vi "execute.vi"(8 "error in (no error)":errorcluster, 9 "DAQ in":refnum<class "GenericComponent.lvclass">, 10 "imaging mode in":refnum<class "GenericComponent.lvclass">, 11 "AdapterDL091214ImagingModeToDAQ in":refnum<class "AdapterDL091214ImagingModeToDAQ.lvclass">) -> (0 "error out":errorcluster, 1 "DAQ out":refnum<class "GenericComponent.lvclass">, 2 "imaging mode out":refnum<class "GenericComponent.lvclass">, 3 "AdapterDL091214ImagingModeToDAQ out":refnum<class "AdapterDL091214ImagingModeToDAQ.lvclass">)   [LabVIEW 2010, in "AdapterDL091214ImagingModeToDAQ.lvclass"]
uses:
  AdapterDL091214ImagingModeToDAQ.lvclass
  common/classes/GenericComponent/GenericComponent/GenericComponent.lvclass
  DAQ/DAQ_MG090622Camera/DAQ_MG090622Camera/DAQ_MG090622Camera.lvclass
  ImagingMode/ImagingModeMG090624Camera/ImagingModeMG090624Camera/ImagingModeMG090624Camera.lvclass
panel:
  # "ScanMode: ImagingModeMG090624Camera \nDAQ: DAQ_MG090622Camera"
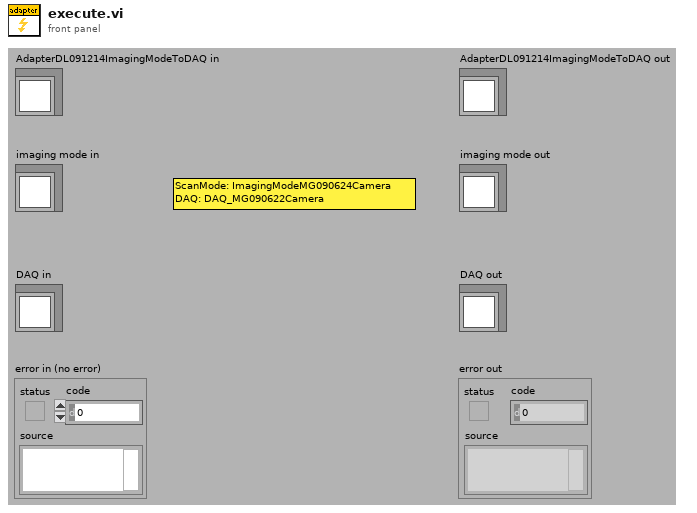
[diagram p1: front panel]
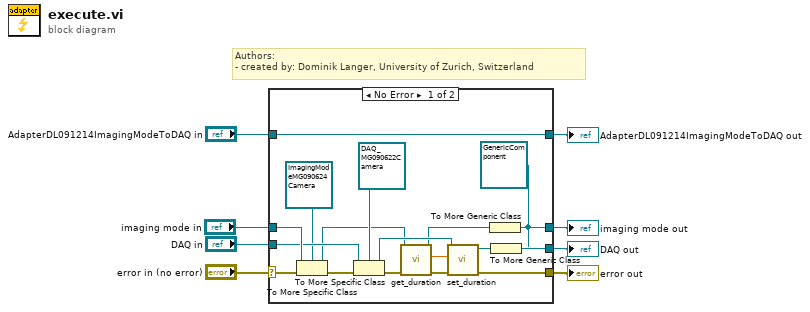
[diagram p0: block diagram]
diagram:
  # "Authors: \n- created by: Dominik Langer, University of Zurich, Switzerland"
  n1 = case shown="No Error" "error in (no error)" {
    selector: "error in (no error)" -> [w25 w29]
    tunnel: "DAQ in" -> [w22 w28]
    tunnel: "imaging mode in" -> [w24 w27]
    tunnel: [w26 w30] -> w4
    tunnel: "AdapterDL091214ImagingModeToDAQ in" -> [w26 w30]
    tunnel: [w16 w29] -> w3
    tunnel: [w19 w28] -> w2
    tunnel: [w17 w27] -> w1
    frame No Error {
      w18 = refnum<class "GenericComponent.lvclass"> refnum ("GenericComponent.lvclass")
      n2 = To More Specific Class(target class=refnum<class "ImagingModeMG090624Camera.lvclass"> refnum ("ImagingModeMG090624Camera.lvclass"), reference=w24, error in=w25) -> (specific class reference=w11:refnum<class "ImagingModeMG090624Camera.lvclass">, error out=w23:errorcluster)
      n3 = To More Specific Class(target class=refnum<class "DAQ_MG090622Camera.lvclass"> refnum ("DAQ_MG090622Camera.lvclass"), reference=w22, error in=w23) -> (specific class reference=w15:refnum<class "DAQ_MG090622Camera.lvclass">, error out=w13:errorcluster)
      n4 = call-dynamic "get_duration.vi"("error in (no error)"=w13, "ScanModeMG090624Camera in"=w11) -> ("error out"=w12:errorcluster, "duration"=w9:dbl[unit], "ScanModeMG090624Camera out"=w10:refnum<class "ImagingModeMG090624Camera.lvclass">)  [unwired: 7 in]
      n5 = call-dynamic "set_duration.vi"("error in (no error)"=w12, "duration"=w9, "DAQ_MG090622Camera in"=w15) -> ("error out"=w16:errorcluster, "DAQ_MG090622Camera out"=w14:refnum<class "DAQ_MG090622Camera.lvclass">)  [unwired: 7 in]
      n6 = To More Generic Class(target class=w18, reference=w10) -> (generic class reference=w17:refnum<class "GenericComponent.lvclass">)
      n7 = To More Generic Class(target class=w18, reference=w14) -> (generic class reference=w19:refnum<class "GenericComponent.lvclass">)
    }
    frame Error {
    }
  }
  "error out" <- w3
  "AdapterDL091214ImagingModeToDAQ out" <- w4
  "imaging mode out" <- w1
  "DAQ out" <- w2
